vi "Corr.vi"(6 "Enum":T1(ring)) -> (2 "H2":dbl format="%#_13g", 3 "H1":dbl format="%#_13g")   [LabVIEW 2019]
uses:
  Global percorso impostazioni.vi
  <vilib>/Utility/file.llb/Read Delimited Spreadsheet (string).vi
  Global CORR.vi
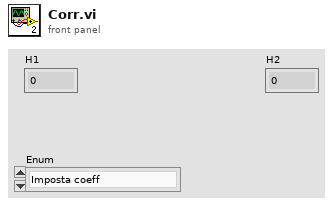
[diagram p1: front panel]
types:
  T1 = enum16{"Imposta coeff", "Coeff NPSH", "Coeff QH", "Leggi coeff"}
  T2 = cluster{"H1 (QH)":dbl, "H2 (QH)":dbl, "H1 (NPSH)":dbl, "H2 (NPSH)":dbl, "Abilita\\disabilita":bool}
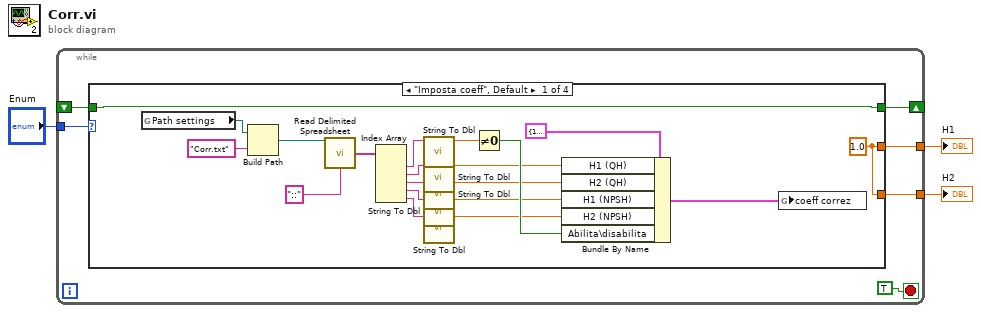
[diagram p0: block diagram]
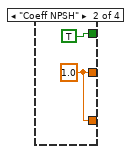
[diagram p2: hidden frame]
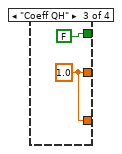
[diagram p3: hidden frame]
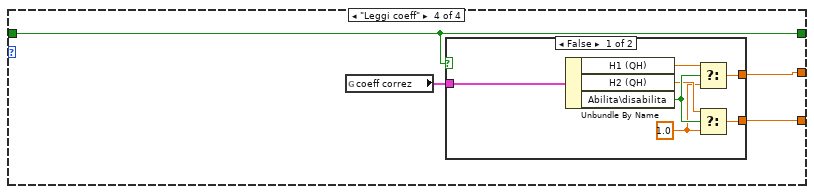
[diagram p4: hidden frame]
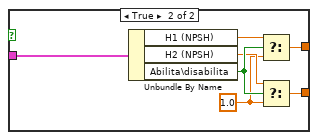
[diagram p5: hidden frame]
diagram:
  n1 = while {
    tunnel: "Enum" -> [w8]
    tunnel: [w7] -> w2
    tunnel: [w6] -> w1
    shift-right: [w5] -> _
    shift-left: _ -> [w4]
    stop <- TRUE stop-if-true
    n2 = case shown="\"Imposta coeff\", Default" w8 {
      tunnel: [w29 w31 w33 w35] -> w7
      tunnel: [w29 w31 w33 w34] -> w6
      tunnel: [w10 TRUE FALSE w36] -> w5
      tunnel: w4 -> [w10 _ _ w36]
      frame "Imposta coeff", Default {
        w29 = 1.0 ("f")
        n3 = global read "Global percorso impostazioni.vi" "Path settings"() -> (w19:path)
        n4 = Build Path(base path=w19, name or relative path="Corr.txt") -> (appended path=w21:path)
        n5 = call-poly <vilib>:"Read Delimited Spreadsheet.vi"("file path (dialog if empty)"=w21, "delimiter (\\t)"="::" ("delimiter (\\t)")) -> ("first row"=w23:string[])  [unwired: 8 in, 5 out]
        n6 = Index Array(array=w23) -> (element #1=w24:string, element #2=w25:string, element #3=w26:string, element #4=w27:string, element #5=w28:string)  [unwired: 5 in]
        n7 = call "String To Dbl.vi"("String"=w24) -> ("Numeric"=w16:dbl)  [unwired: 10 in]
        n8 = call "String To Dbl.vi"("String"=w25) -> ("Numeric"=w14:dbl)  [unwired: 10 in]
        n9 = call "String To Dbl.vi"("String"=w26) -> ("Numeric"=w13:dbl)  [unwired: 10 in]
        n10 = call "String To Dbl.vi"("String"=w27) -> ("Numeric"=w12:dbl)  [unwired: 10 in]
        n11 = call "String To Dbl.vi"("String"=w28) -> ("Numeric"=w11:dbl)  [unwired: 10 in]
        n12 = Not Equal To 0?(x=w16) -> (x != 0?=w15:bool)
        n13 = Bundle By Name(cluster=T2 {"H1 (QH)"=1.0, "H2 (QH)"=1.0, "H1 (NPSH)"=1.0, "H2 (NPSH)"=1.0, "Abilita\\disabilita"=FALSE} ("coeff correz"), "H1 (QH)"=w14, "H2 (QH)"=w13, "H1 (NPSH)"=w12, "H2 (NPSH)"=w11, "Abilita\\disabilita"=w15) -> (w18:T2)
        n14 = global write "Global CORR.vi" "coeff correz"(w18) -> ()
      }
      frame "Coeff NPSH" {
        w31 = 1.0 ("f")
      }
      frame "Coeff QH" {
        w33 = 1.0 ("f")
      }
      frame "Leggi coeff" {
        n15 = global read "Global CORR.vi" "coeff correz"() -> (w37:T2)
        n16 = case shown="False" w36 {
          tunnel: w37 -> [w44 w51]
          tunnel: [w39 w46] -> w35
          tunnel: [w38 w45] -> w34
          frame False {
            w40 = 1.0 ("f")
            n17 = Unbundle By Name(w44) -> ("H1 (QH)"=w42:dbl, "H2 (QH)"=w41:dbl, "Abilita\\disabilita"=w43:bool)
            n18 = Select(t=w42, s=w43, f=w40) -> (s? t:f=w39:dbl)
            n19 = Select(t=w41, s=w43, f=w40) -> (s? t:f=w38:dbl)
          }
          frame True {
            w47 = 1.0 ("f")
            n20 = Unbundle By Name(w51) -> ("H1 (NPSH)"=w49:dbl, "H2 (NPSH)"=w48:dbl, "Abilita\\disabilita"=w50:bool)
            n21 = Select(t=w49, s=w50, f=w47) -> (s? t:f=w46:dbl)
            n22 = Select(t=w48, s=w50, f=w47) -> (s? t:f=w45:dbl)
          }
        }
      }
    }
  }
  "H1" <- w2
  "H2" <- w1
